vi "main.vi"() -> ()   [LabVIEW 2023]
uses:
  <vilib>/Rock Robotics/WPI/ThirdParty/JAS_Junk/TrajLib/Trajectory_Library.lvlib
panel:
  out "Rise Time Condition":bool
  out "Overshoot Condition":bool
  in  "stop":bool
  in  "ArmAngle_Goal_Deg":dbl=60.0 format="%#_13g"
  out "ArmAngle_Gauge_Deg":dbl(knob) scale=180.0..-180.0
  out "ArmSpeed_RadPerSec":dbl format="%#_3g"
  out "ArmAngle_Deg":dbl format="%#_3g"
  out "XY Graph":cluster{"Y":dbl[], "Y":dbl[]}[](graph)
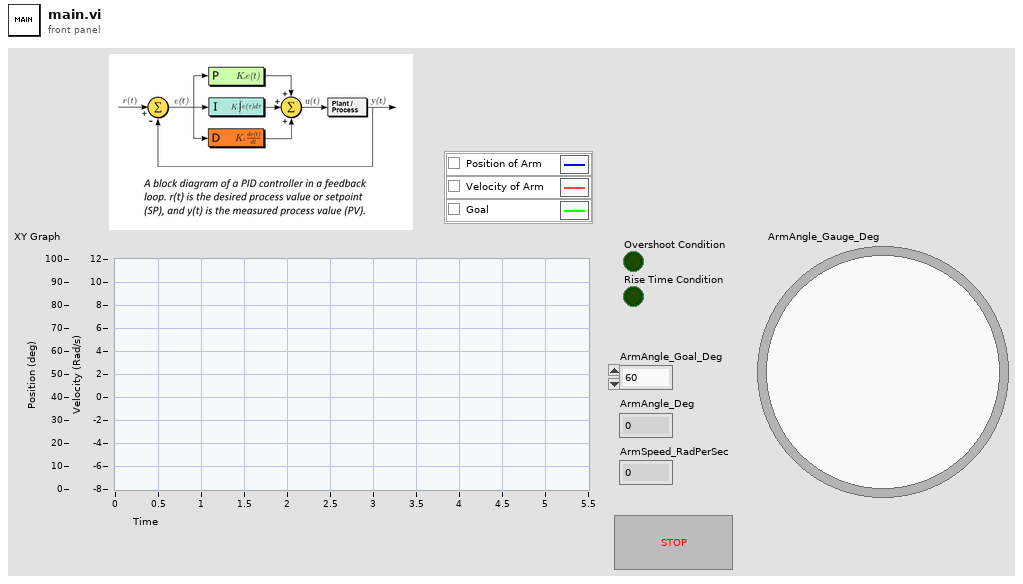
[diagram p1: front panel]
types:
  T1 = cluster{"proportional gain (Kp)":dbl, "integral gain (Ki)":dbl, "derivative gain (Kd)":dbl}
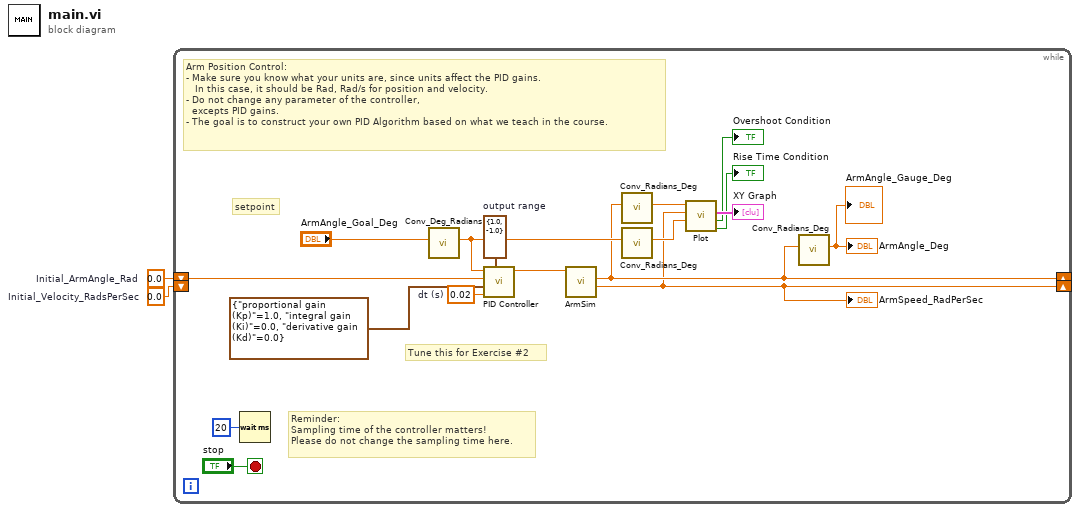
[diagram p0: block diagram]
diagram:
  w1 = 0.0  # Initial_Velocity_RadsPerSec
  w2 = 0.0  # Initial_ArmAngle_Rad
  n1 = while {
    shift-right: [w8] -> _
    shift-left: w2 -> [w14]
    shift-right: [w6] -> _
    shift-left: w1 -> [_]
    stop <- "stop" stop-if-true
    w16 = 0.02  # dt (s)
    w18 = cluster{"high":dbl, "low":dbl} {"high"=1.0, "low"=-1.0}  # output range
    # "Tune this for Exercise #2"
    # "setpoint"
    # "Arm Position Control: \n- Make sure you know what your units are, since units affect the PID gains.\n   In this case, it should be Rad, Rad/s for position and velocity.\n- Do not change any parameter of the controller, \n  excepts PID gains.\n- The goal is to construct your own PID Algorithm based on what we teach in the course."
    # "Reminder:\nSampling time of the controller matters!\nPlease do not change the sampling time here."
    n2 = Wait (ms)(milliseconds to wait=u32 20) -> ()  [unwired: 1 out]
    n3 = call <vilib>:"Conv_Deg_Radians.vi"("Degress"="ArmAngle_Goal_Deg") -> ("Radians"=w9:dbl)  [unwired: 10 in]
    n4 = call "PID Controller.vi"("output range"=w18, "dt (s)"=w16, "PID gains"=T1 {"proportional gain (Kp)"=1.0, "integral gain (Ki)"=0.0, "derivative gain (Kd)"=0.0}, "process variable"=w14, "setpoint"=w9) -> ("output"=w15:dbl)  [unwired: 4 in, 2 out]
    n5 = call "ArmSim.vi"("Motor Dmd"=w15) -> ("Velocity_RadsPerSec"=w6:dbl, "ArmAngle_Rad"=w8:dbl)  [unwired: 9 in]
    "ArmSpeed_RadPerSec" <- w6
    n6 = call <vilib>:"Conv_Radians_Deg.vi"("Radians"=w8) -> ("Degrees"=w12:dbl)  [unwired: 10 in]
    n7 = call <vilib>:"Conv_Radians_Deg.vi"("Radians"=w9) -> ("Degrees"=w10:dbl)  [unwired: 10 in]
    n8 = call "Plot.vi"("Position_Goal_Deg"=w10, "Velocity_RadPerSec"=w6, "Position_Deg"=w12) -> ("Rise Time Condition"=→"Rise Time Condition":bool, "Overshoot Condition"=→"Overshoot Condition":bool, "XY Graph"=→"XY Graph":cluster{"Y":dbl[], "Y":dbl[]}[])  [unwired: 6 in]
    n9 = call <vilib>:"Conv_Radians_Deg.vi"("Radians"=w8) -> ("Degrees"=→"ArmAngle_Deg" →"ArmAngle_Gauge_Deg":dbl)  [unwired: 10 in]
  }
